vi "Create Waveform.vi"(4 "sampling info":cluster{"Fs":dbl, "#s":dbl}={"Fs"=100000000.0, "#s"=4000.0}, 7 "signal type":T1(ring), 8 "error in (no error)":errorcluster, 9 "phase":dbl format="%.2p", 10 "amplitude":dbl=1.0 format="%0.2p", 11 "frequency":dbl=10.0 format="%0.2p") -> (0 "error out":errorcluster, 2 "Output Waveform Size":u32, 3 "Output Waveform (V)":waveform(dbl))   [LabVIEW 2018, in "GettingStarted_5785_Host.lvlib"]
uses:
  GettingStarted_5785_Host.lvlib
  <vilib>/measure/NI_MABase.lvlib
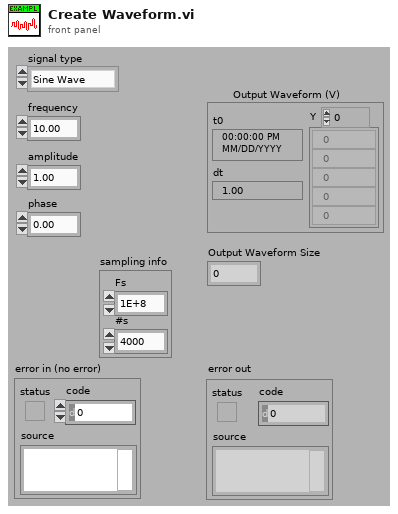
[diagram p1: front panel]
types:
  T1 = enum16{"Sine Wave", "Triangle Wave", "Square Wave", "Sawtooth Wave"}
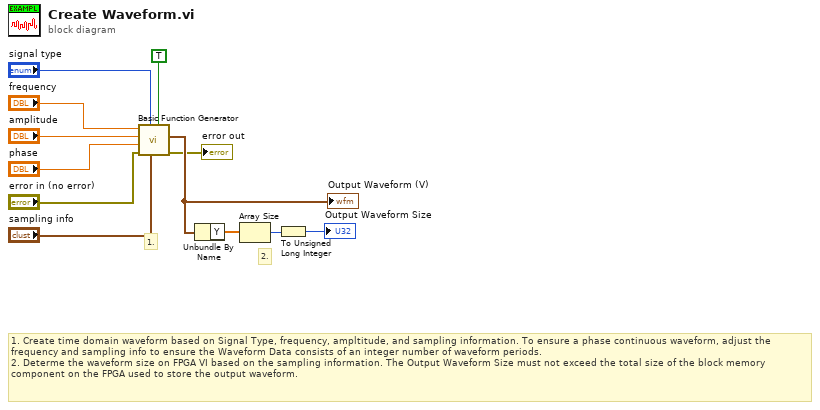
[diagram p0: block diagram]
diagram:
  # "2."
  # "1. Create time domain waveform based on Signal Type, frequency, ampltitude, and sampling information. To ensure a phase continuous waveform, adjust the frequency and sampling info to ensure the Waveform Data consists of an integer number of waveform periods.\n2. Determe the waveform size on FPGA VI based on the sampling information. The Output Waveform Size must not exceed the total size of the block memory component on the FPGA used to store the output waveform."
  # "1."
  n1 = call <vilib>:"Basic Function Generator.vi"("reset signal"=TRUE, "sampling info"="sampling info", "signal type"="signal type", "error in (no error)"="error in (no error)", "phase"="phase", "amplitude"="amplitude", "frequency"="frequency") -> ("error out"=→"error out":errorcluster, "signal out"=w11:waveform(dbl))  [unwired: 2 in, 1 out]
  "Output Waveform (V)" <- w11
  n2 = Unbundle By Name(w11) -> ("Y"=w9:dbl[])
  n3 = Array Size(array=w9) -> (size(s)=w12:i32)
  n4 = To Unsigned Long Integer(number=w12) -> (unsigned 32bit integer=→"Output Waveform Size":u32)
